vi "Square Negate.vi"(1 "x":dbl) -> (0 "x脖":dbl)   [LabVIEW 2012]
doc: "Squares a number and negates it according to input value."
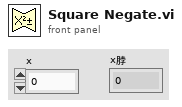
[diagram p1: front panel]
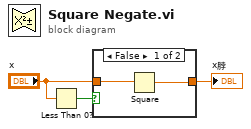
[diagram p0: block diagram]
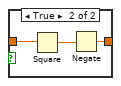
[diagram p2: hidden frame]
diagram:
  n1 = Less Than 0?(x="x") -> (x < 0?=w2:bool)
  n2 = case shown="False" w2 {
    tunnel: "x" -> [w5 w7]
    tunnel: [w4 w8] -> w3
    frame False {
      n3 = Square(x=w5) -> (x^2=w4:dbl)
    }
    frame True {
      n4 = Square(x=w7) -> (x^2=w6:dbl)
      n5 = Negate(x=w6) -> (-x=w8:dbl)
    }
  }
  "x脖" <- w3
